vi "Untitled 9.vi"() -> ()   [LabVIEW 2020]
uses:
  <vilib>/DAQmx/read.llb/DAQmx Read (Analog 1D Wfm NChan NSamp).vi
  <vilib>/DAQmx/miscellaneous.llb/DAQmx Fill In Error Info.vi
panel:
  in  "stop":bool
  out "data":waveform(dbl)[](graph)
  in  "DAQmx Task Name":refnum<k21>="NSamplesAI"
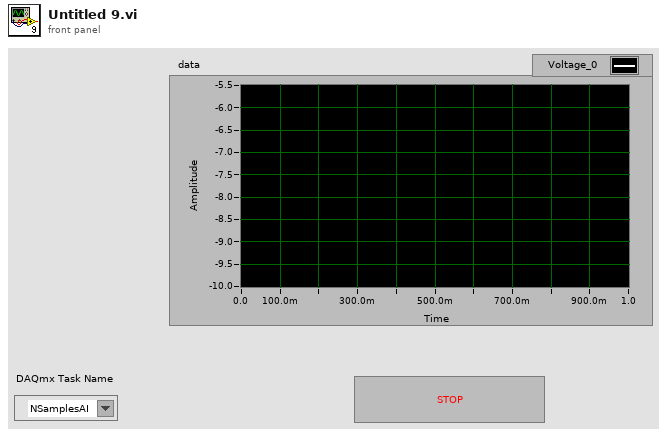
[diagram p1: front panel]
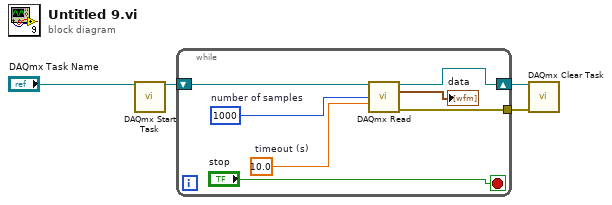
[diagram p0: block diagram]
diagram:
  n1 = call <vilib>:"DAQmx Start Task.vi"("task/channels in"="DAQmx Task Name") -> ("task out"=w1:refnum<k21>)  [unwired: 13 in, 1 out]
  n2 = while {
    tunnel: [w8] -> w4
    shift-right: [w7] -> w3
    shift-left: w1 -> [w6]
    stop <- "stop" stop-if-true
    w9 = 10.0  # timeout (s)
    w10 = 1000  # number of samples
    n3 = call-poly <vilib>:"DAQmx Read.vi"("task/channels in"=w6, "number of samples per channel"=w10, "timeout"=w9) -> ("task out"=w7:refnum<k21>, "data"=→"data":waveform(dbl)[], "error out"=w8:errorcluster)  [unwired: 10 in]
  }
  n4 = call <vilib>:"DAQmx Clear Task.vi"("task in"=w3, "error in"=w4) -> ()  [unwired: 13 in, 1 out]
